vi "Asynchronous - Detect Change in Array U16.vi"(8 "Error (in)":errorcluster, 10 "Data (in)":u16[](array[numeric])) -> (0 "Error (out)":errorcluster, 1 "Indexes":i32[](array[numeric]), 2 "Data (out)":u16[](array[numeric]))   [LabVIEW 2019, in "Ballard MIL-1553 Engine.lvlib"]
uses:
  Ballard MIL-1553 Engine.lvlib
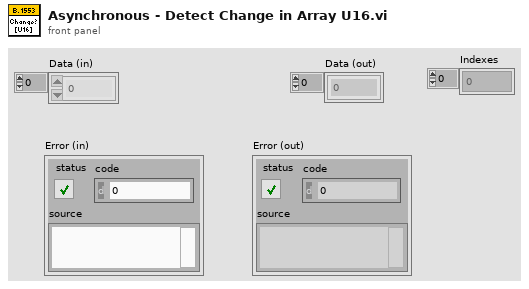
[diagram p1: front panel]
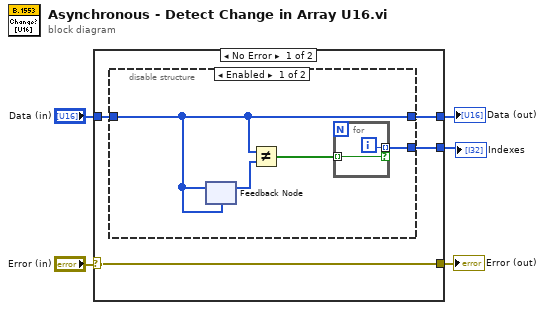
[diagram p0: block diagram]
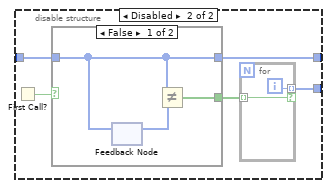
[diagram p2: hidden frame]
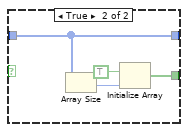
[diagram p3: hidden frame]
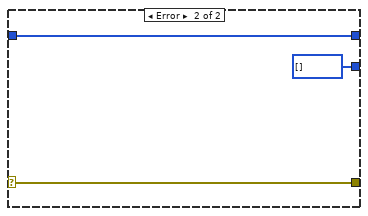
[diagram p4: hidden frame]
diagram:
  n1 = case shown="No Error" "Error (in)" {
    selector: "Error (in)" -> [w7 w32]
    tunnel: "Data (in)" -> [w9 w31]
    tunnel: [w8 w31] -> w4
    tunnel: [w7 w32] -> w2
    tunnel: [w6 i32[] []] -> w1
    frame No Error {
      n2 = disable-structure shown="Enabled" {
        disable-tunnel: w9 -> [w10 w20]
        disable-tunnel: [w10 w18] -> w8
        disable-tunnel: [w12 w16] -> w6
        frame Enabled {
          n3 = feedback #1(w10) -> (w11:u16[])
          n4 = feedback-in #1(w10) -> ()
          n5 = Not Equal?(x=w10, y=w11) -> (x != y?=w13:bool[])
          n6 = for {
            tunnel: w13 -> [w15] mode=indexing
            tunnel: [w14] -> w12 mode=indexing if=w15
            i -> [w14]
          }
        }
        frame Disabled {
          n7 = First Call?() -> (First Call?: T/F=w17:bool)
          n8 = case shown="False" w17 {
            tunnel: w20 -> [w21 w27]
            tunnel: [w22 w24] -> w19
            tunnel: [w21 w27] -> w18
            frame False {
              n9 = feedback #2() -> (w23:u16[])  [unwired: 1 in]
              n10 = feedback-in #2(w21) -> ()
              n11 = Not Equal?(x=w21, y=w23) -> (x != y?=w22:bool[])
            }
            frame True {
              n12 = Array Size(array=w27) -> (size(s)=w26:i32)
              n13 = Initialize Array(TRUE, w26) -> (w24:bool[])
            }
          }
          n14 = for {
            tunnel: w19 -> [w28] mode=indexing
            tunnel: [w29] -> w16 mode=indexing if=w28
            i -> [w29]
          }
        }
      }
    }
    frame Error {
    }
  }
  "Error (out)" <- w2
  "Data (out)" <- w4
  "Indexes" <- w1
